vi "ToCowlAngle.vi"(1 "Initial Angle(Degrees)":dbl, 2 "Input(Encoder Units)":dbl) -> (0 "Angle(Degrees)":dbl)   [LabVIEW 2019]
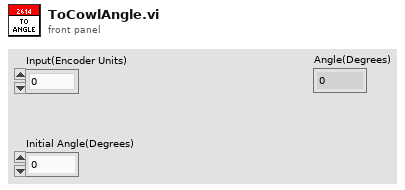
[diagram p1: front panel]
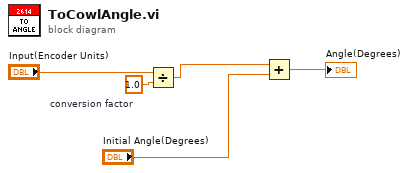
[diagram p0: block diagram]
diagram:
  w2 = 1.0  # conversion factor
  n1 = Divide(x="Input(Encoder Units)", y=w2) -> (x/y=w1:dbl)
  n2 = Add(x=w1, y="Initial Angle(Degrees)") -> (x+y=→"Angle(Degrees)":dbl)
